vi "Home.vi"(8 "error in (no error)":errorcluster, 10 "shutdown":refnum<user-event>, 11 "Modules":T4) -> (0 "error out":errorcluster)   [LabVIEW 2025]
uses:
  Controls/refresh button 2.ctl
  Controls/Test list.ctl
  Classes/Solenoid/Solenoid Selector.ctl
  <vilib>/Handler Framework/CmdQueue/Enqueue Single.vi
  <vilib>/Handler Framework/Handler Framework.lvlib
panel:
  out "error out 2":errorcluster
  in  "Part Number":T1
  in  "Run Tests":bool
  in  "Test Selection":T2
  in  "Refresh":T3
  # "Home"
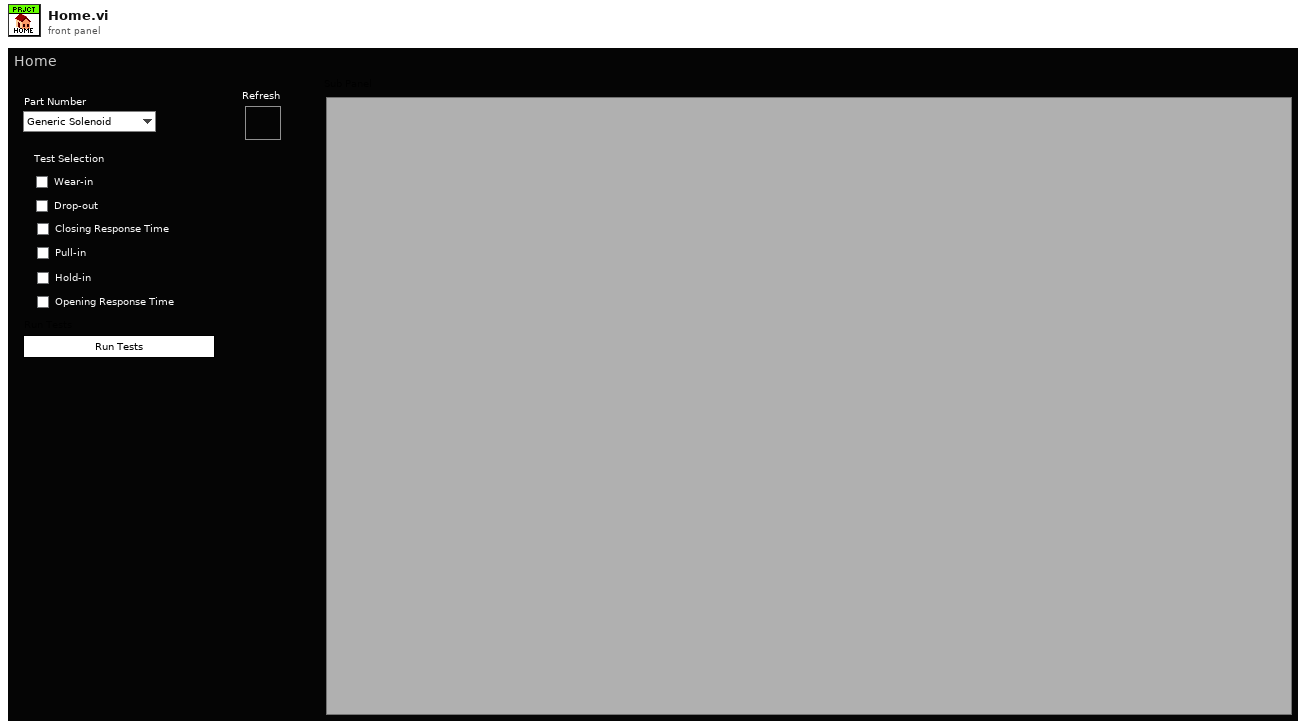
[diagram p1: front panel]
types:
  T1 = typedef "Solenoid Selector.ctl" = enum16{"Generic Solenoid", "EVI-79"}
  T2 = typedef "Test list.ctl" = cluster{"Wear-in":bool, "Drop-out":bool, "Closing Response Time":bool, "Pull-in":bool, "Hold-in":bool, "Opening Response Time":bool}
  T3 = typedef "refresh button 2.ctl" = bool
  T4 = cluster{"Module IDs":i32[], "Module Names":string[]}
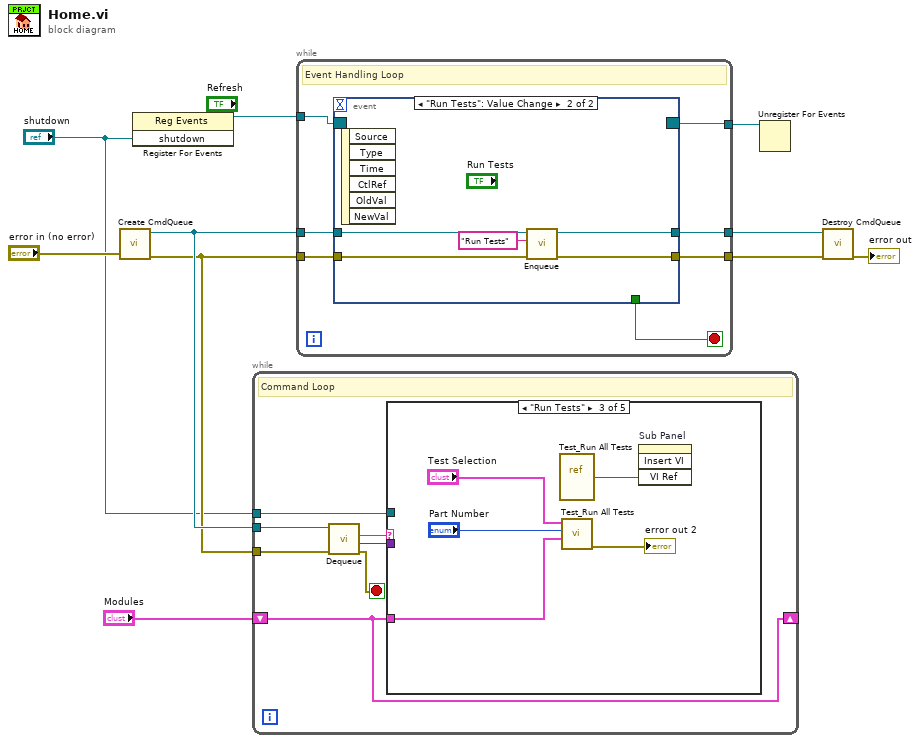
[diagram p0: block diagram]
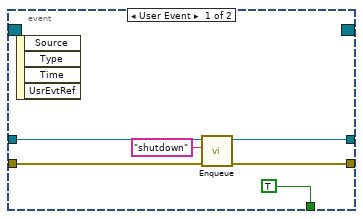
[diagram p6: hidden frame]
diagram:
  n1 = call <vilib>:"Create CmdQueue.vi"("error in (no error)"="error in (no error)") -> ("error out"=w7:errorcluster, "CmdQueue out"=w8:refnum<queue>)  [unwired: 9 in]
  n2 = register-events("shutdown") -> (reference out=w6:refnum<event-registration>)  [unwired: 2 in, 1 out]
  n3 = while {
    tunnel: w8 -> [w17]
    tunnel: w7 -> [w13]
    tunnel: "shutdown" -> [w12]
    shift-right: [w11] -> _
    shift-left: "Modules" -> [w11]
    stop <- w14 stop-if-true
    # "Command Loop"
    n4 = call <vilib>:"Dequeue.vi"("error in (no error)"=w13, "CmdQueue in"=w17) -> ("error out"=w14:errorcluster, "value"=w15:variant, "cmd"=w16:string)  [unwired: 5 in, 2 out]
    n5 = case shown="\"Run Tests\"" w16 {
      tunnel: w15 -> [_ _ _ _ _]
      tunnel: w12 -> [_ _ _ _ _]
      tunnel: w11 -> [_ _ w20 _ _]
      frame "False", Default {
      }
      frame "init" {
      }
      frame "Run Tests" {
        n6 = vi-ref "Test_Run All Tests.vi"() -> (w18:refnum<vi>)
        n7 = call "Test_Run All Tests.vi"("Modules"=w20, "Part Number"="Part Number", "Test Selection"="Test Selection") -> ("error out"=→"error out 2":errorcluster)  [unwired: 8 in]
        n8 = invoke on="Sub Panel" class="SubPnl" method="Insert VI"("VI Ref"=w18) -> ()  [unwired: 3 in, 4 out]
      }
      frame "shutdown" {
      }
      frame "refresh" {
      }
    }
  }
  n9 = while {
    tunnel: w8 -> [w29]
    tunnel: [w28] -> w10
    tunnel: w7 -> [w27]
    tunnel: [w26] -> w9
    tunnel: w6 -> [w24]
    tunnel: [w23] -> w5
    stop <- w25 stop-if-true
    # "Event Handling Loop"
    n10 = event shown="[1] \"Run Tests\": Value Change" {
      selector: w24 -> [_ _]
      dyn-events: [_ _] -> w23
      timeout: _ -> [_ _]
      tunnel: w29 -> [w35 w40]
      tunnel: [w34 w39] -> w28
      tunnel: w27 -> [w33 w38]
      tunnel: [w32 w37] -> w26
      tunnel: [TRUE ("Discard?") _] -> w25
      event User Event {
        n11 = event-data() -> ()  [unwired: 1 in, 4 out]
        n12 = call-poly <vilib>:"Enqueue.vi"("error in (no error)"=w33, "Command"="shutdown", "CmdQueue in"=w35) -> ("error out"=w32:errorcluster, "CmdQueue out"=w34:refnum<queue>)  [unwired: 7 in]
      }
      event "Run Tests": Value Change {
        n13 = event-data() -> ()  [unwired: 1 in, 6 out]
        n14 = call-poly <vilib>:"Enqueue.vi"("error in (no error)"=w38, "Command"="Run Tests", "CmdQueue in"=w40) -> ("error out"=w37:errorcluster, "CmdQueue out"=w39:refnum<queue>)  [unwired: 7 in]
      }
    }
  }
  n15 = Unregister For Events(event registration refnum=w5) -> ()  [unwired: 1 in, 1 out]
  n16 = call <vilib>:"Destroy CmdQueue.vi"("error in (no error)"=w9, "CmdQueue in"=w10) -> ("error out"=→"error out":errorcluster)  [unwired: 9 in]
